vi "Directionater.vi"(9 "Y In":dbl, 11 "X In":dbl) -> (1 "Y":dbl, 2 "Rotation":dbl)   [LabVIEW 2016]
uses:
  <vilib>/Analysis/baseanly.llb/A x Vector.vi
  <vilib>/Analysis/NI_AALBase.lvlib
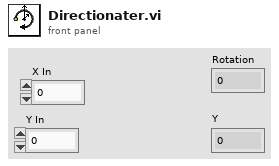
[diagram p1: front panel]
types:
  T1 = cluster{"Yaw":dbl, "Roll":dbl, "Pitch":dbl, "Heading":dbl, "Fused Heading":dbl}
  T2 = typedef "NI_Matrix.lvlib/RealMatrix.ctl" = dbl[][]
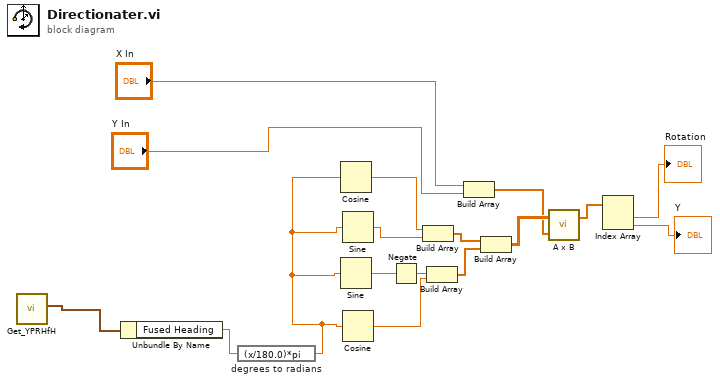
[diagram p0: block diagram]
diagram:
  n1 = call <vilib>:"Get_YPRHfH.vi"() -> ("YRPHfH"=w2:T1)  [unwired: 11 in]
  n2 = Unbundle By Name(w2) -> ("Fused Heading"=w1:dbl)
  n3 = expression code="(x/180.0)*pi" "degrees to radians"(w1) -> (w9:dbl)
  n4 = Cosine(x=w9) -> (cos(x)=w15:dbl)
  n5 = Sine(x=w9) -> (sin(x)=w14:dbl)
  n6 = Sine(x=w9) -> (sin(x)=w8:dbl)
  n7 = Cosine(x=w9) -> (cos(x)=w13:dbl)
  n8 = Negate(x=w14) -> (-x=w7:dbl)
  n9 = Build Array(w15, w8) -> (w16:dbl[])
  n10 = Build Array(w7, w13) -> (w17:dbl[])
  n11 = Build Array("X In", "Y In") -> (w11:dbl[])
  n12 = Build Array(w16, w17) -> (w12:T2)
  n13 = call-poly <vilib>:"A x B.vi"("Vector"=w11, "A"=w12) -> ("A x Vector"=w10:dbl[])  [unwired: 1 out]
  n14 = Index Array(array=w10) -> (element #1=→"Rotation":dbl, element #2=→"Y":dbl)  [unwired: 2 in]
